vi "VI_deciamteData.vi"(9 "Factor":i32, 10 "DataPoints":cluster{"Time":dbl, "Value":dbl}[](array[cluster])) -> (3 "Array":cluster{"Time":dbl, "Value":dbl}[](array[cluster]))   [LabVIEW 2020]
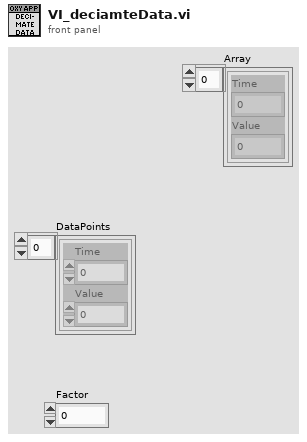
[diagram p1: front panel]
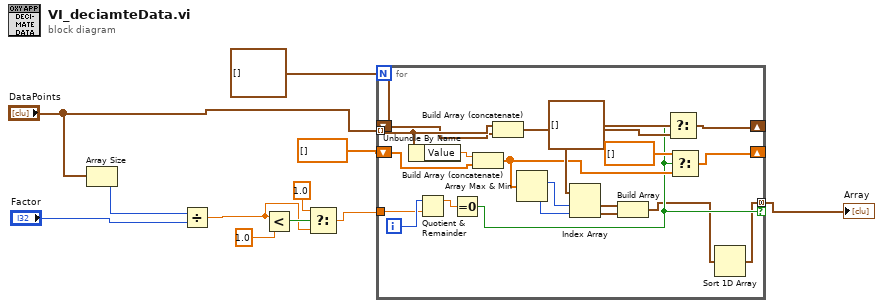
[diagram p0: block diagram]
diagram:
  n1 = Array Size(array="DataPoints") -> (size(s)=w2:i32)
  n2 = Divide(x=w2, y="Factor") -> (x/y=w1:dbl)
  n3 = Less?(x=w1, y=1.0) -> (x < y?=w8:bool)
  n4 = Select(t=1.0, s=w8, f=w1) -> (s? t:f=w9:dbl)
  n5 = for {
    tunnel: "DataPoints" -> [w26] mode=indexing
    shift-right: [w20] -> _
    shift-left: dbl[] [] ("t") -> [w30]
    tunnel: w9 -> [w28]
    shift-right: [w21] -> _
    shift-left: cluster{"Time":dbl, "Value":dbl}[] [] ("t") -> [w25]
    tunnel: [w12] -> w4 mode=concatenating if=w14
    i -> [w29]
    n6 = Unbundle By Name(w26) -> ("Value"=w31:dbl)
    n7 = Quotient & Remainder(x=w29, y=w28) -> (x-y*floor(x/y)=w27:dbl)  [unwired: 1 out]
    n8 = Equal To 0?(x=w27) -> (x = 0?=w14:bool)
    n9 = Build Array (concatenate)(w31, w30) -> (w19:dbl[])
    n10 = Build Array (concatenate)(w26, w25) -> (w22:cluster{"Time":dbl, "Value":dbl}[])
    n11 = Array Max & Min(array=w19) -> (max index (indices)=w24:i32, min index (indices)=w23:i32)  [unwired: 2 out]
    n12 = Index Array(array=w22, index #1=w24, index #2=w23) -> (element #1=w16:cluster{"Time":dbl, "Value":dbl}, element #2=w15:cluster{"Time":dbl, "Value":dbl})
    n13 = Build Array(w16, w15) -> (w13:cluster{"Time":dbl, "Value":dbl}[])
    n14 = Select(t=cluster{"Time":dbl, "Value":dbl}[] [], s=w14, f=w22) -> (s? t:f=w21:cluster{"Time":dbl, "Value":dbl}[])
    n15 = Select(t=dbl[] [], s=w14, f=w19) -> (s? t:f=w20:dbl[])
    n16 = Sort 1D Array(array=w13) -> (sorted array=w12:cluster{"Time":dbl, "Value":dbl}[])
  }
  "Array" <- w4
